vi "Example_LowLevelZoom.vi"() -> ()   [LabVIEW 2020, in "LcPictureBox.lvclass"]
uses:
  LcPictureBox.lvclass
  CallBacks/MouseWheelInfo.ctl
  System.Drawing
  CallBackVIs/CallBack_MouseWheel.vi
  System.Windows.Forms
panel:
  in  "PictureBox":refnum<k24>(container)
types:
  T1 = typedef "LcPictureBox.lvclass/MouseWheelInfo.ctl" = cluster{"X":i32, "Y":i32, "Button":i32, "Delta":i32, "X(raw)":i32, "Y(raw)":i32}
  T2 = cluster{"reference out":refnum<class "LcPictureBox.lvclass">, "MouseInfo":refnum<user-event>}
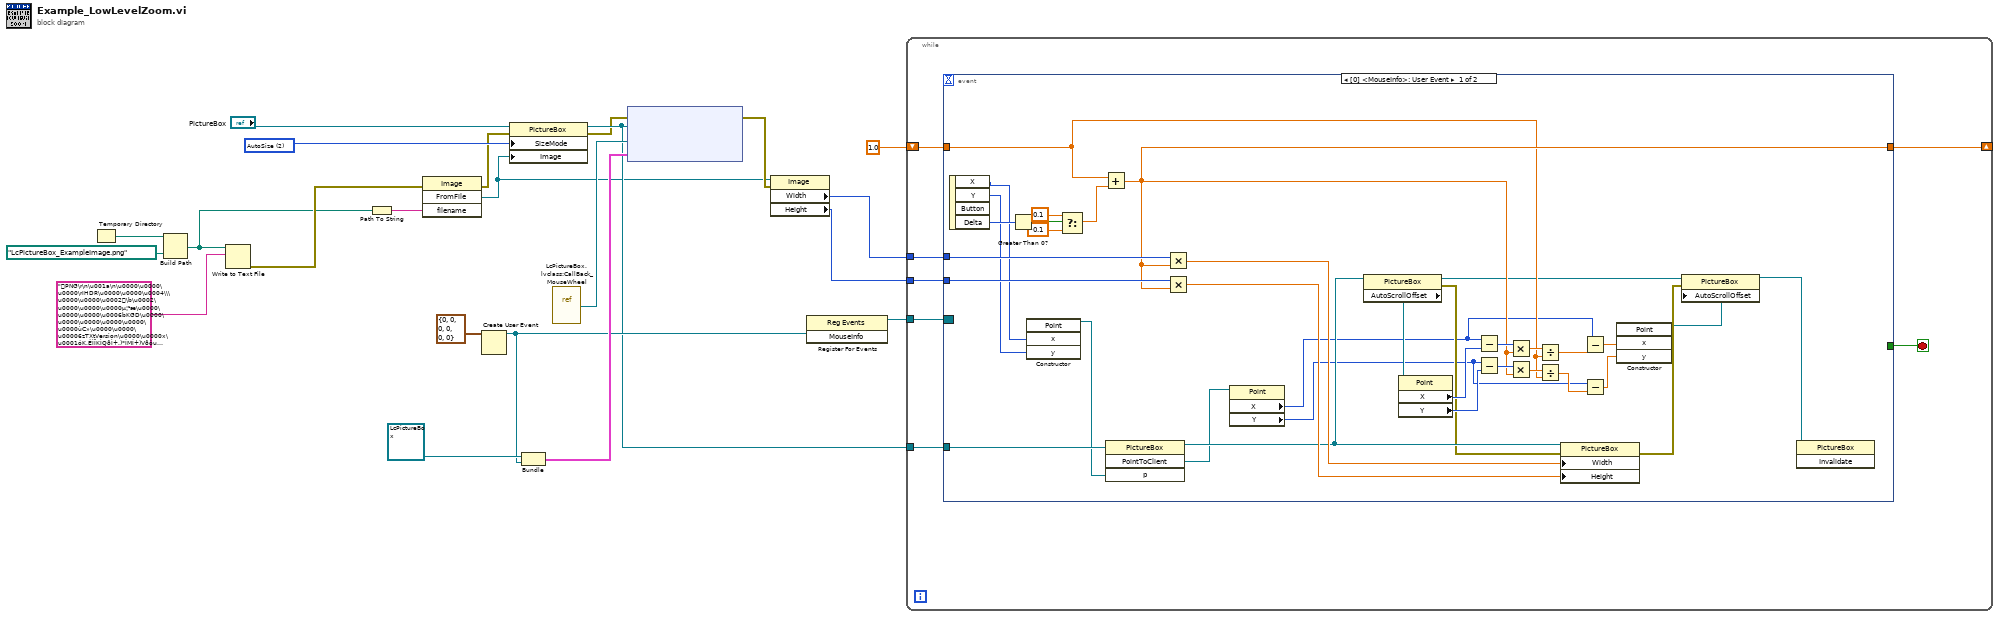
[diagram p0: block diagram]
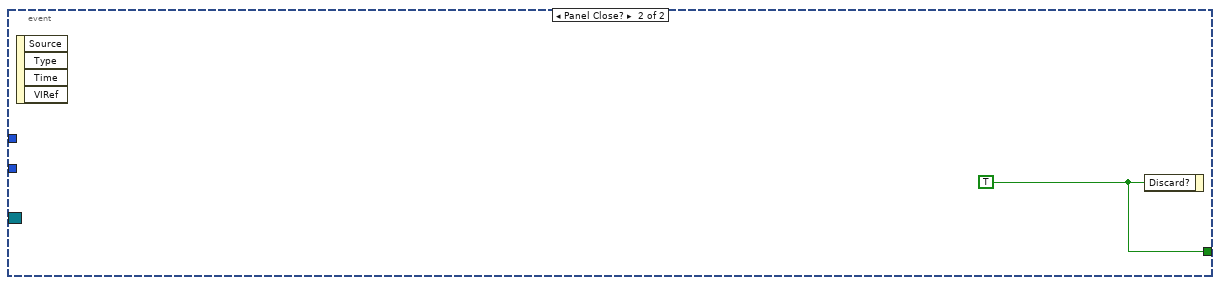
[diagram p2: hidden frame]
diagram:
  w21 = 2 items=["Normal", "StretchImage", "AutoSize", "CenterImage", "Zoom"] ("AutoSize")
  n1 = Temporary Directory() -> (w5:path)
  n2 = Build Path(base path=w5, name or relative path=path "LcPictureBox_ExampleImage.png") -> (appended path=w1:path)
  n3 = Write to Text File(file (use dialog)=w1, text="PNG\r\n\u001a\n\u0000\u0000\u0000\rIHDR\u0000\u0000\u0004\\\u0000\u0000\u0002\b\u0002\u0000\u0000\u0000µ¦¹æ\u0000\u0000\u0000\u0006bKGD\u0000\u0000\u0000\u0000\u0000\u0000ùC»\u0000\u0000\u00006zTXtVersion\u0000\u0000x\u0001óK,ÉÌÏKÌQðÌ+.)*ÍMÍ+)Vðôu\fT\bË,\u0006Ê(Xèé\u0019\u0000\u0000\u0012y\fýZÐ|y\u0000\u0000\u0000\u000ftEXtNI Image Type\u00004ÉÁÏz\u0000\u0000 \u0000IDATx\u0001ì½\u0007X\u001bWÚþo÷¿ov³iNqbÇ+\u0018Lï½&$!¡$Ô\u0010¢*è½÷nlãÞ°Á»1îÆ½÷\u001a×¸÷n¾[L¢(É²ëlòf_gëÎ¹F3Ã\fç7÷ó<ç\u001dgG\u001fädçü½\\í5dëêüÜ\\ìÔR\u000fþ¤£¹»Ó/\u0012ÉÕÑÍÅ8´£­¦\u001cí­!\u0007;+;\u001b\u000bÈÆÚÜÚÊÌÒÜ\u0018²0327545621246Ô72Ð\u001b3rÖx=/\u000f¿´ô\u0002&G\u0014\u0014\u0016\u001b\u0015*\u000eð\u0017J¥aá1ñ<±, 0X\u0012\"\u0017ÉÂE²ÐÀ aPª#\u000bñðe0ø\u0001Þ~LqH\u0018FìÝÜC¢b\u0018\\¾$4Îá9<¤!r\u000e_\"\u0004{}¿\u001c®õ÷\u000fF|òé\u0004\u001f\u001fÙ¶-§6m>±¾÷ðªu{º×îíX³gNçÖ¹+wv÷Z¶ýÈÆÃgrêlÝ=\u0002#£¢þB,\"8£¸$)¿0¿¢êÞËWÐýþ~èAÿ/o<{vóùó+\u000f\u001f^ú\u0014í\u001b7ö<½rË¶Ùí\u001dÓ\u0017·u¬íYÞ³ióÞ\u0003GÎ_<yéúów\u001e>Ù¹nãÌ%Í\u000b,\\¾zï©ów½zÜßÿ...") -> (error out=w2:errorcluster)  [unwired: 2 in, 2 out]
  n4 = Path To String(path=w1) -> (string=w20:string)
  n5 = invoke class="Image" method="FromFile"(error in=w2, "filename"=w20) -> (error out=w9:errorcluster, "FromFile"=w6:refnum<k24>)  [unwired: 2 in, 2 out]
  n6 = Create User Event(user event datatype=T1 {"X"=0, "Y"=0, "Button"=0, "Delta"=0, "X(raw)"=0, "Y(raw)"=0} ("MouseInfo")) -> (user event=w15:refnum<user-event>)  [unwired: 1 in, 1 out]
  n7 = property class="PictureBox"(reference="PictureBox", error in=w9, "SizeMode"=w21, "Image"=w6) -> (reference out=w12:refnum<k24>, error out=w8:errorcluster)
  n8 = Bundle("reference out"=refnum<class "LcPictureBox.lvclass"> refnum, "MouseInfo"=w15) -> (w16:T2)  [unwired: 1 in]
  n9 = vi-ref "LcPictureBox.lvclass:CallBack_MouseWheel.vi"() -> ("vi reference"=w17:refnum<vi>)
  n10 = node(w8, w12, w17, w16) -> (w7:errorcluster)  [unwired: 1 in, 1 out]
  n11 = property class="Image"(reference=w6, error in=w7) -> ("Width"=w11:i32, "Height"=w10:i32)  [unwired: 2 out]
  n12 = register-events(w15) -> (reference out=w14:refnum<event-registration>)  [unwired: 2 in, 1 out]
  n13 = while {
    tunnel: w14 -> [w29]
    shift-right: [w27] -> _
    shift-left: 1.0 -> [w28]
    tunnel: w12 -> [w26]
    tunnel: w11 -> [w25]
    tunnel: w10 -> [w24]
    stop <- w23 stop-if-true
    n14 = event shown="[0] <MouseInfo>: User Event" {
      selector: w29 -> [_ _]
      dyn-events: _ -> [_ _]
      timeout: _ -> [_ _]
      tunnel: w28 -> [w44 _]
      tunnel: [w47 _] -> w27
      tunnel: w26 -> [w59 _]
      tunnel: w25 -> [w57 _]
      tunnel: w24 -> [w56 _]
      tunnel: [_ w65] -> w23
      event User Event {
        n15 = event-data() -> ("X"=w33:i32, "Y"=w31:i32, "Delta"=w64:i32)  [unwired: 1 in, 1 out]
        n16 = Greater Than 0?(x=w64) -> (x > 0?=w63:bool)
        n17 = constructor class="Point"("x"=w33, "y"=w31) -> (reference out=w58:refnum<k24>)  [unwired: 3 in, 4 out]
        n18 = Select(t=0.1, s=w63, f=-0.1 ("t")) -> (s? t:f=w60:dbl)
        n19 = Add(x=w44, y=w60) -> (x+y=w47:dbl)
        n20 = invoke class="PictureBox" method="PointToClient"(reference=w59, "p"=w58) -> (reference out=w53:refnum<k24>, "PointToClient"=w34:refnum<k24>)  [unwired: 2 in, 2 out]
        n21 = Multiply(x=w57, y=w47) -> (x*y=w55:dbl)
        n22 = Multiply(x=w56, y=w47) -> (x*y=w54:dbl)
        n23 = property class="Point"(reference=w34) -> ("X"=w32:i32, "Y"=w30:i32)  [unwired: 1 in, 2 out]
        n24 = property class="PictureBox"(reference=w53) -> (reference out=w37:refnum<k24>, error out=w39:errorcluster, "AutoScrollOffset"=w52:refnum<k24>)  [unwired: 1 in]
        n25 = property class="Point"(reference=w52) -> ("X"=w51:i32, "Y"=w50:i32)  [unwired: 1 in, 2 out]
        n26 = Subtract(x=w32, y=w51) -> (x-y=w49:i32)
        n27 = Subtract(x=w30, y=w50) -> (x-y=w48:i32)
        n28 = Multiply(x=w49, y=w47) -> (x*y=w46:dbl)
        n29 = Multiply(x=w48, y=w47) -> (x*y=w45:dbl)
        n30 = Divide(x=w46, y=w44) -> (x/y=w43:dbl)
        n31 = Divide(x=w45, y=w44) -> (x/y=w42:dbl)
        n32 = property class="PictureBox"(reference=w53, error in=w39, "Width"=w55, "Height"=w54) -> (error out=w38:errorcluster)  [unwired: 1 out]
        n33 = Subtract(x=w32, y=w43) -> (x-y=w41:dbl)
        n34 = Subtract(x=w30, y=w42) -> (x-y=w40:dbl)
        n35 = constructor class="Point"("x"=w41, "y"=w40) -> (reference out=w36:refnum<k24>)  [unwired: 3 in, 4 out]
        n36 = property class="PictureBox"(reference=w37, error in=w38, "AutoScrollOffset"=w36) -> (reference out=w35:refnum<k24>)  [unwired: 1 out]
        n37 = invoke class="PictureBox" method="Invalidate"(reference=w35) -> ()  [unwired: 2 in, 3 out]
      }
      event Panel Close? {
        w65 = TRUE ("Discard?")
        n38 = event-data() -> ()  [unwired: 1 in, 4 out]
        n39 = event-data("Discard?"=w65) -> ()  [unwired: 1 in, 1 out]
      }
    }
  }
